vi "Is OOT.vi"(1 "Comp":T1, 2 "Result":dbl=10.99 format="%.3f", 3 "UL":dbl=11.0 format="%.3f", 4 "LL":dbl=9.0 format="%.3f") -> (0 "OOT":bool)   [LabVIEW 2010]
doc: "Compare value to absolute nominal limits (inclusive).\nIf the lower limit is greater than the upper limit, then the limits are swapped.\nIf error or enable is FALSE, then result is NaN and status is FAIL."
uses:
  Comparison Control.ctl
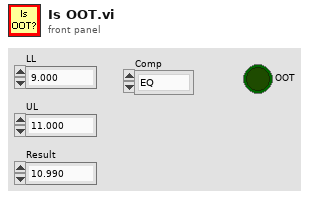
[diagram p1: front panel]
types:
  T1 = typedef "Comparison Control.ctl" = enum16{"EQ", "GE", "GELE", "GELT", "GT", "GTLE", "GTLT", "LE", "LT", "NE", "None"}
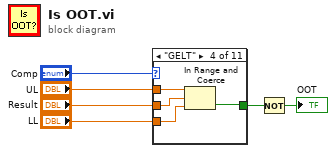
[diagram p0: block diagram]
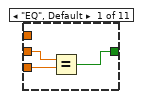
[diagram p2: hidden frame]
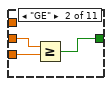
[diagram p3: hidden frame]
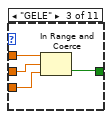
[diagram p4: hidden frame]
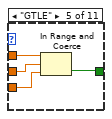
[diagram p5: hidden frame]
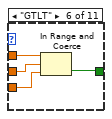
[diagram p6: hidden frame]
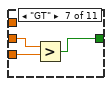
[diagram p7: hidden frame]
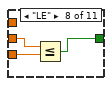
[diagram p8: hidden frame]
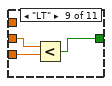
[diagram p9: hidden frame]
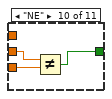
[diagram p10: hidden frame]
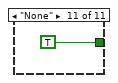
[diagram p11: hidden frame]
diagram:
  n1 = case shown="\"GELT\"" "Comp" {
    tunnel: "LL" -> [w9 w12 w14 w18 w22 w26 w31 w34 w37 w40 _]
    tunnel: "UL" -> [_ _ w16 w20 w24 w28 _ _ _ _ _]
    tunnel: "Result" -> [w8 w11 w15 w19 w23 w27 w30 w33 w36 w39 _]
    tunnel: [w7 w10 w13 w17 w21 w25 w29 w32 w35 w38 TRUE] -> w2
    frame "EQ", Default {
      n2 = Equal?(x=w8, y=w9) -> (x = y?=w7:bool)
    }
    frame "GE" {
      n3 = Greater Or Equal?(x=w11, y=w12) -> (x >= y?=w10:bool)
    }
    frame "GELE" {
      n4 = In Range and Coerce(upper limit=w16, x=w15, lower limit=w14) -> (In Range?=w13:bool)  [unwired: 1 out]
    }
    frame "GELT" {
      n5 = In Range and Coerce(upper limit=w20, x=w19, lower limit=w18) -> (In Range?=w17:bool)  [unwired: 1 out]
    }
    frame "GTLE" {
      n6 = In Range and Coerce(upper limit=w24, x=w23, lower limit=w22) -> (In Range?=w21:bool)  [unwired: 1 out]
    }
    frame "GTLT" {
      n7 = In Range and Coerce(upper limit=w28, x=w27, lower limit=w26) -> (In Range?=w25:bool)  [unwired: 1 out]
    }
    frame "GT" {
      n8 = Greater?(x=w30, y=w31) -> (0:w29:bool)
    }
    frame "LE" {
      n9 = Less Or Equal?(x=w33, y=w34) -> (x <= y?=w32:bool)
    }
    frame "LT" {
      n10 = Less?(x=w36, y=w37) -> (x < y?=w35:bool)
    }
    frame "NE" {
      n11 = Not Equal?(x=w39, y=w40) -> (x != y?=w38:bool)
    }
    frame "None" {
    }
  }
  n12 = Not(x=w2) -> (.not. x?=→"OOT":bool)
